vi "Write Data to VS Engine.vi"(8 "error in":errorcluster, 10 "Write to VS Engine FIFO":refnum<k33>, 11 "Channel Pairs":T2 {"Chan Refs" format="%.0x"}) -> (0 "error out":errorcluster, 2 "Read Occured":bool, 3 "Channel Pairs Out":T2 {"Chan Refs" format="%.0x"})   [LabVIEW 2015, in "Diagnostics Addon Engine.lvlib" / "Inline Async API.lvlib"]
uses:
  Inline Async API.lvlib
  <vilib>/NI Veristand/Custom Device API/Data Reference.ctl
  <vilib>/NI Veristand/Custom Device API/Global Data Refs.vi
  <vilib>/NI Veristand/Custom Device API/Custom Device API.lvlib
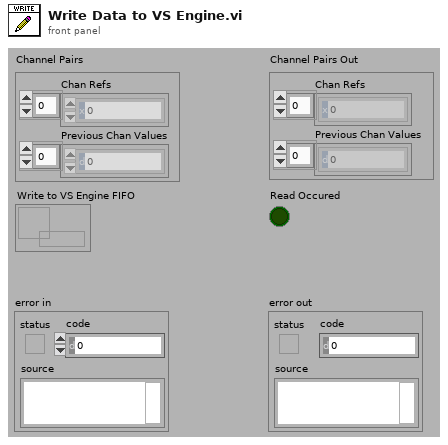
[diagram p1: front panel]
types:
  T1 = typedef "Custom Device API.lvlib/Data Reference.ctl" = i32
  T2 = cluster{"Chan Refs":T1[], "Previous Chan Values":dbl[]}
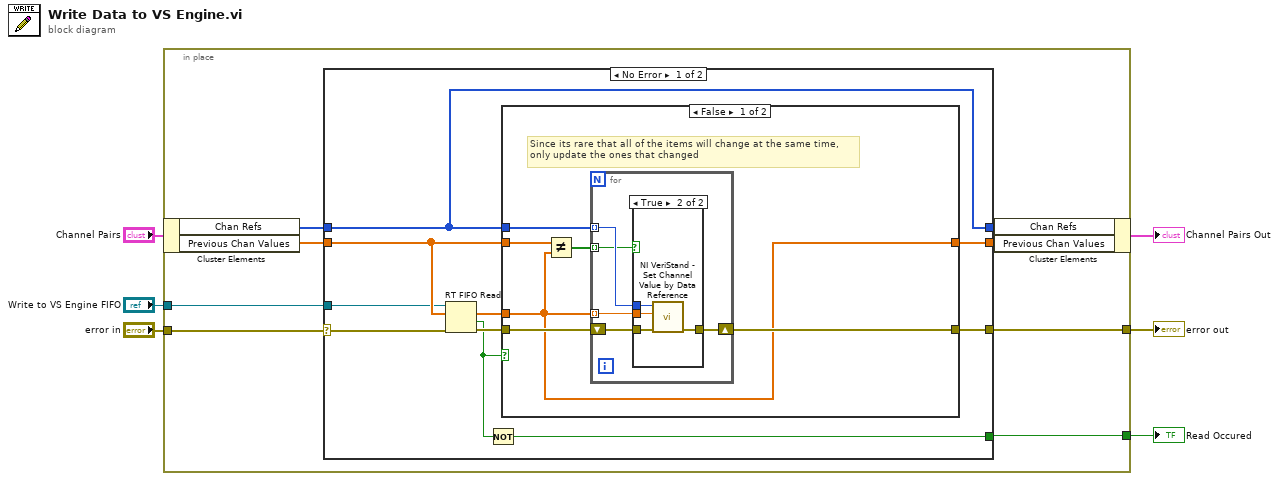
[diagram p0: block diagram]
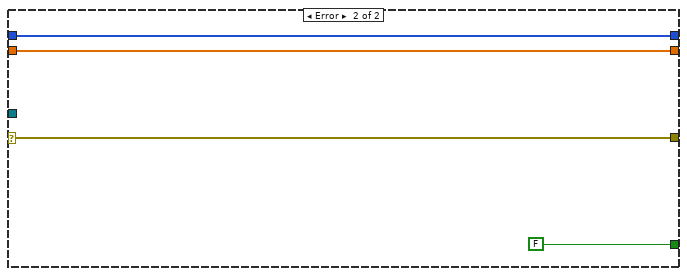
[diagram p4: hidden frame]
diagram:
  n1 = in-place {
    in-place-border: [w14] -> w6
    in-place-border: [w13] -> w5
    in-place-border: "error in" -> [w8]
    in-place-border: "Write to VS Engine FIFO" -> [w7]
    n2 = in-place-cluster #1("Channel Pairs") -> ("Chan Refs"=w12:T1[], "Previous Chan Values"=w11:dbl[])
    n3 = case shown="No Error" w8 {
      selector: w8 -> [w21 w46]
      tunnel: [w24 w46] -> w14
      tunnel: [w17 w44] -> w10
      tunnel: [w19 FALSE ("C Read Occured?")] -> w13
      tunnel: w12 -> [w16 w43]
      tunnel: w11 -> [w18 w44]
      tunnel: [w16 w43] -> w9
      tunnel: w7 -> [w15 _]
      frame No Error {
        n4 = RT FIFO Read(0:w15, 1:w18, 3:w21) -> (9:w22:dbl[], 10:w20:bool, 11:w23:errorcluster)  [unwired: 1 in, 2 out]
        n5 = Not(x=w20) -> (.not. x?=w19:bool)
        n6 = case shown="False" w20 {
          tunnel: w23 -> [w30 w42]
          tunnel: w22 -> [w25 _]
          tunnel: [w29 w42] -> w24
          tunnel: [w25 w41] -> w17
          tunnel: w16 -> [w28 _]
          tunnel: w18 -> [w26 w41]
          frame False {
            # "Since its rare that all of the items will change at the same time,\nonly update the ones that changed"
            n7 = Not Equal?(x=w26, y=w25) -> (x != y?=w27:bool[])
            n8 = for {
              shift-right: [w35] -> w29
              shift-left: w30 -> [w34]
              tunnel: w27 -> [w31] mode=indexing
              tunnel: w25 -> [w33] mode=indexing
              tunnel: w28 -> [w32] mode=indexing
              n9 = case shown="True" w31 {
                tunnel: w33 -> [_ w37]
                tunnel: [w36 w39] -> w35
                tunnel: w34 -> [w36 w40]
                tunnel: w32 -> [_ w38]
                frame False {
                }
                frame True {
                  n10 = call <vilib>:"NI VeriStand - Set Channel Value by Data Reference.vi"("error in (no error)"=w40, "Value"=w37, "Data Reference in"=w38) -> ("error out"=w39:errorcluster)  [unwired: 8 in]
                }
              }
            }
          }
          frame True {
          }
        }
      }
      frame Error {
      }
    }
    n11 = in-place-cluster #1("Chan Refs"=w9, "Previous Chan Values"=w10) -> (→"Channel Pairs Out":T2)
  }
  "error out" <- w6
  "Read Occured" <- w5
